vi "LVProjectShortcut_InitProperties.vi"(8 "error in":errorcluster, 11 "Wizard":T1) -> (0 "error out":errorcluster)   [LabVIEW 2017]
uses:
  <resource>/Framework/Providers/API/ItemRef.ctl
  <resource>/Framework/Providers/API/mxLvSetBooleanProperty.vi
  <resource>/Framework/Providers/API/mxLvSetStringProperty.vi
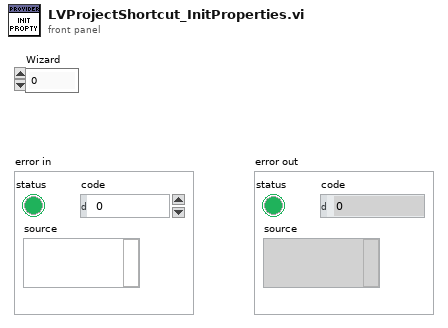
[diagram p1: front panel]
types:
  T1 = typedef "ItemRef.ctl" = u64
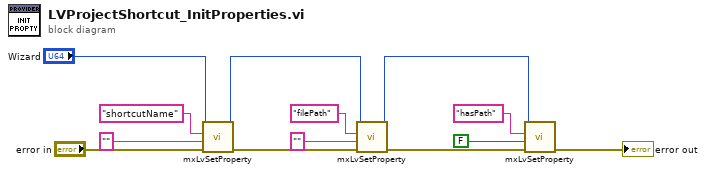
[diagram p0: block diagram]
diagram:
  n1 = call-poly <resource>:"mxLvSetProperty.vi"("error in"="error in", "Value (\"\")"="" ("Value (\"\")"), "Tag"="shortcutName", "Item"="Wizard") -> ("error out"=w9:errorcluster, "Item"=w6:T1)  [unwired: 6 in]
  n2 = call-poly <resource>:"mxLvSetProperty.vi"("error in"=w9, "Value (\"\")"="" ("Value (\"\")"), "Tag"="filePath", "Item"=w6) -> ("error out"=w2:errorcluster, "Item"=w1:T1)  [unwired: 6 in]
  n3 = call-poly <resource>:"mxLvSetProperty.vi"("error in"=w2, "Value (F)"=FALSE, "Tag"="hasPath", "Item"=w1) -> ("error out"=→"error out":errorcluster)  [unwired: 6 in, 1 out]
